vi "nominal ingest tabular set timestamp epoch.vi"(8 "error in (no error)":errorcluster, 9 "time_unit":i32, 10 "column":string, 11 "staging":i32) -> (0 "error out":errorcluster, 3 "function return":i32)   [LabVIEW 2020, in "client.lvlib"]
doc: "int32_t nominal_ingest_tabular_set_timestamp_epoch(int32_t staging,\n const char *column,\n int32_t time_unit);"
uses:
  client.lvlib
  bin/nominalClient_64.dll
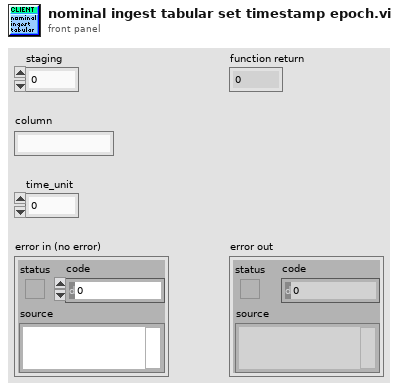
[diagram p1: front panel]
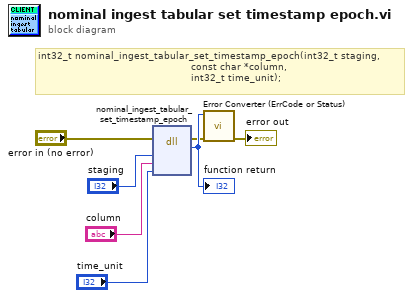
[diagram p0: block diagram]
diagram:
  # "int32_t nominal_ingest_tabular_set_timestamp_epoch(int32_t staging,\n                                                   const char *column,\n                                                   int32_t time_unit);"
  n1 = dll-call lib="C:/code/labview-client-rs/lv_src/bin/nominalClient_*.*" fn="nominal_ingest_tabular_set_timestamp_epoch"(error in="error in (no error)", "staging"="staging", "column"="column", "time_unit"="time_unit") -> (error out=w2:errorcluster, w7:i32)  [unwired: 5 in, 1 out]
  "function return" <- w7
  n2 = call "Error Converter (ErrCode or Status).vi"("error in (no error)"=w2, "error code"=w7) -> ("error out"=→"error out":errorcluster)  [unwired: 9 in]
